vi "Enumerate CB.vi"(7 "Data":string, 8 "error in (no error)":errorcluster, 11 "IP Connection in":refnum<class "IP Connection.lvclass">) -> (0 "error out":errorcluster, 2 "Enumerate CB":T1, 3 "IP Connection out":refnum<class "IP Connection.lvclass">)   [LabVIEW 2011, in "Tinkerforge.lvlib" / "IP Connection.lvclass"]
doc: "This VI decodes the <B>Enumerate Callback</B>."
uses:
  IP Connection.lvclass
  Type Definitions/Enumerate CB.ctl
  IP Connection.lvclass/IP Connection.ctl
  Tinkerforge.lvlib
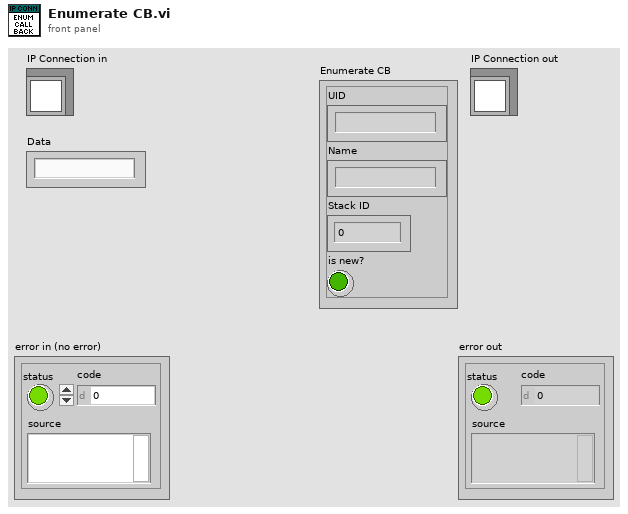
[diagram p1: front panel]
types:
  T1 = typedef "Tinkerforge.lvlib/IP Connection.lvclass/Enumerate CB.ctl" = cluster{"UID":string, "Name":string, "Stack ID":u8, "is new?":bool}
  T2 = enum16{"big-endian, network order", "native, host order", "little-endian"}
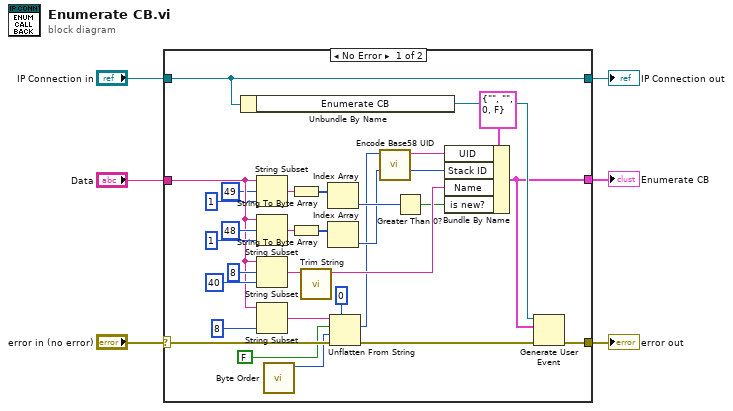
[diagram p0: block diagram]
diagram:
  n1 = case shown="No Error" "error in (no error)" {
    selector: "error in (no error)" -> [w35 w38]
    tunnel: [w11 w38] -> w5
    tunnel: [w13 w37] -> w3
    tunnel: "IP Connection in" -> [w13 w37]
    tunnel: "Data" -> [w25 _]
    tunnel: [w9 _] -> w1
    frame No Error {
      n2 = Unbundle By Name(w13) -> ("Enumerate CB"=w10:refnum<user-event>)
      n3 = String Subset(string=w25, offset (0)=49, length (rest)=1 ("length (rest)")) -> (substring=w22:string)
      n4 = String Subset(string=w25, offset (0)=48, length (rest)=1 ("length (rest)")) -> (substring=w16:string)
      n5 = String Subset(string=w25, offset (0)=8, length (rest)=40 ("length (rest)")) -> (substring=w18:string)
      n6 = String Subset(string=w25, length (rest)=8 ("length (rest)")) -> (substring=w32:string)  [unwired: 1 in]
      n7 = call "Byte Order.vi"() -> ("byte order (2:little-endian)"=w34:T2)  [unwired: 11 in]
      n8 = String To Byte Array(string=w22) -> (unsigned byte array=w21:u8[])
      n9 = String To Byte Array(string=w16) -> (unsigned byte array=w17:u8[])
      n10 = call "Trim String.vi"("String"=w18) -> ("trimmed string"=w26:string)  [unwired: 10 in]
      n11 = Index Array(array=w21) -> (element=w20:u8)  [unwired: 1 in]
      n12 = Index Array(array=w17) -> (element=w15:u8)  [unwired: 1 in]
      n13 = Unflatten From String(type=u64 0, binary string=w32, data includes array or string size? (T)=FALSE, byte order (0:big-endian, network order)=w34, error in (no error)=w35) -> (value=w8:u64, error out=w12:errorcluster)  [unwired: 1 out]
      n14 = call "Encode Base58 UID.vi"("UID"=w8) -> ("Base58 UID"=w7:string)  [unwired: 9 in, 1 out]
      n15 = Greater Than 0?(x=w20) -> (x > 0?=w14:bool)
      n16 = Bundle By Name(cluster=T1 {"UID"="", "Name"="", "Stack ID"=0, "is new?"=FALSE} ("Enumerate CB"), "UID"=w7, "Stack ID"=w15, "Name"=w26, "is new?"=w14) -> (w9:T1)
      n17 = Generate User Event(user event=w10, event data cluster=w9, error in=w12) -> (error out=w11:errorcluster)  [unwired: 1 out]
    }
    frame Error {
    }
  }
  "error out" <- w5
  "IP Connection out" <- w3
  "Enumerate CB" <- w1
